vi "PPMS_FreqMeas.vi"(6 "error in (no error)":errorcluster, 7 "Index":i8) -> (0 "error out":errorcluster, 1 "MeasConfig":T1={"Tiempo (sec)"=10.0, "Campo X (T)"=0.025, "Campo Y (T)"=10.0, "Campo Z (T)"=0.025, "Temperatura (K)"=0.025, "Start Frequency (Hz)"=100000.0, "Stop Frequency (Hz)"=1000000.0, "IF Bandwidth"=25.0, "Sweep time(s)"=25.0, "Meas Points"=201, "Power Level (0.0)"=-40.0} {"Campo Z (T)" format="%^.2e"; "Campo Y (T)" format="%^.2e"; "Sweep time(s)" format="%^.2g"; "Temperatura (K)" format="%^.2e"; "Campo X (T)" format="%^.2e"; "Tiempo (sec)" format="%^.2g"; "Start Frequency (Hz)" format="%^.2e"; "IF Bandwidth" format="%^.2e"; "Power Level (0.0)" format="%^.2g"}, 2 "resulting string 1":string="Spectrum from 1.0E+1 Hz to 1.0E+1 Hz, Bandwidth 1.00 Hz, 10 points, Power 10.00 dB", 3 "Cancelled?":bool=TRUE)   [LabVIEW 2017]
doc: "Use this template to create a dialog box. This template polls the state of the buttons on the front panel and does not use events. Use the Dialog Using Events template (not available in Base package) to create a dialog box with event handling."
uses:
  RohdeSchwarz ZNB MeasConfig.ctl
panel:
  in  "Power Level (dB)":dbl=-20.0 format="%.2f"
  in  "Start Frequency (Hz)":dbl=10000000.0 format="%.2p"
  in  "Stop Frequency (Hz)":dbl=10000000000.0 format="%.2p"
  out "MODE":i32(ring) items=["SET&MEAS", "SCAN", "MEASURE ENA3G"]
  in  "IF Bandwidth (Hz)":dbl=50000.0 format="%.2p"
  in  "# Points (2..1601)":u16=5000
  in  "Cancel":bool
  in  "OK":bool
  # "Nov 2020 V1.2  a-sslcdms"
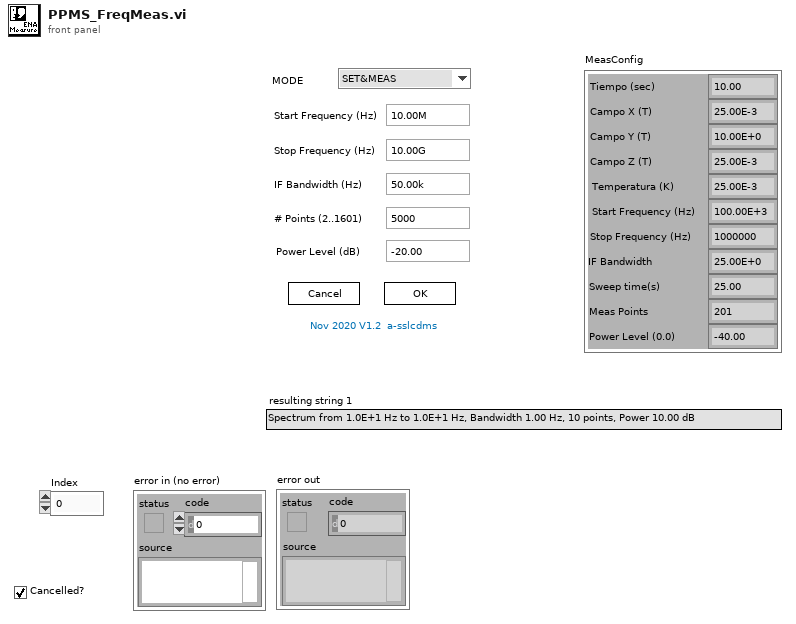
[diagram p1: front panel]
types:
  T1 = typedef "RohdeSchwarz ZNB MeasConfig.ctl" = cluster{"Tiempo (sec)":dbl, "Campo X (T)":dbl, "Campo Y (T)":dbl, "Campo Z (T)":dbl, "Temperatura (K)":dbl, "Start Frequency (Hz)":dbl, "Stop Frequency (Hz)":dbl, "IF Bandwidth":dbl, "Sweep time(s)":dbl, "Meas Points":i32, "Power Level (0.0)":dbl}
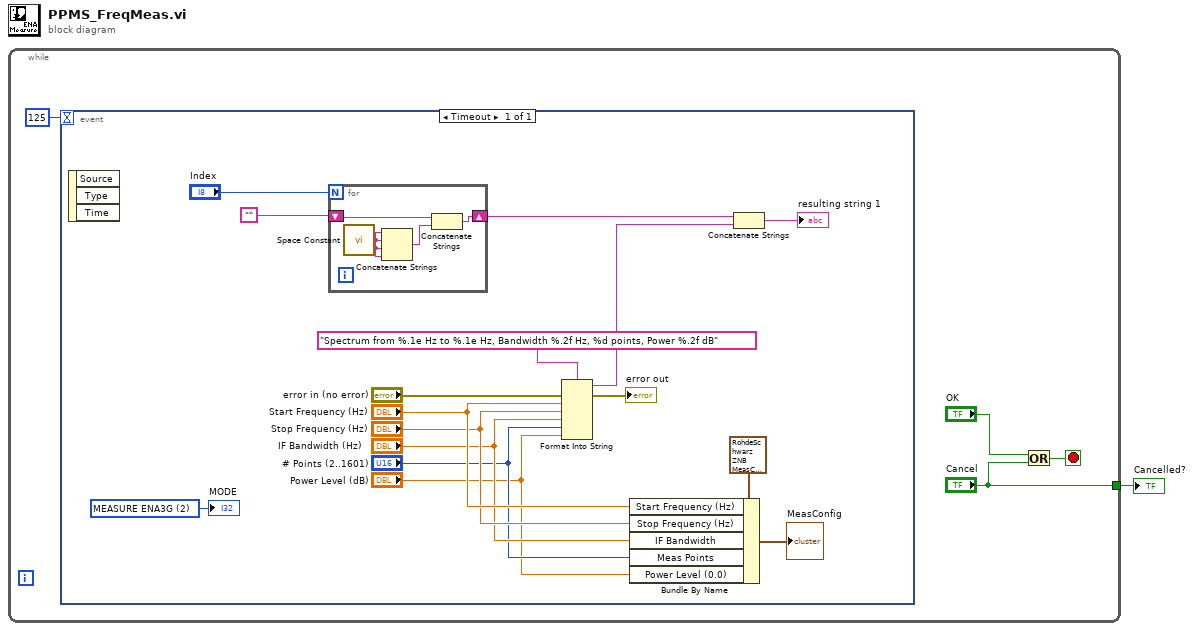
[diagram p0: block diagram]
diagram:
  n1 = while {
    tunnel: ["Cancel"] -> w1
    stop <- w4 stop-if-true
    n2 = event shown="[0] Timeout" {
      selector: _ -> [_]
      dyn-events: _ -> [_]
      timeout: 125 -> [_]
      event Timeout {
        w6 = 2 items=["SET&MEAS", "SCAN", "MEASURE ENA3G"] ("MODE")
        n3 = event-data() -> ()  [unwired: 1 in, 3 out]
        n4 = for {
          N: "Index" -> [_]
          shift-right: [w24] -> w21
          shift-left: "" -> [w23]
          n5 = call <vilib>:"Space Constant.vi"() -> ("String"=w22:string)
          n6 = Concatenate Strings(w22, w22, w22, w22) -> (w25:string)
          n7 = Concatenate Strings(w23, w25) -> (w24:string)
        }
        n8 = Format Into String(format string="Spectrum from %.1e Hz to %.1e Hz, Bandwidth %.2f Hz, %d points, Power %.2f dB", error in="error in (no error)", "Start Frequency (Hz)", "Stop Frequency (Hz)", "IF Bandwidth (Hz)", "# Points (2..1601)", "Power Level (dB)") -> (resulting string=w19:string, error out=→"error out":errorcluster)  [unwired: 1 in]
        n9 = Bundle By Name(cluster=T1 {"Tiempo (sec)"=10.0, "Campo X (T)"=0.025, "Campo Y (T)"=10.0, "Campo Z (T)"=0.025, "Temperatura (K)"=0.025, "Start Frequency (Hz)"=100000.0, "Stop Frequency (Hz)"=1000000.0, "IF Bandwidth"=25.0, "Sweep time(s)"=25.0, "Meas Points"=201, "Power Level (0.0)"=-40.0} ("MeasConfig"), "Start Frequency (Hz)"="Start Frequency (Hz)", "Stop Frequency (Hz)"="Stop Frequency (Hz)", "IF Bandwidth"="IF Bandwidth (Hz)", "Meas Points"="# Points (2..1601)", "Power Level (0.0)"="Power Level (dB)") -> (→"MeasConfig":T1)
        n10 = Concatenate Strings(w21, w19) -> (→"resulting string 1":string)
        "MODE" <- w6
      }
    }
    n11 = Or(x="OK", y="Cancel") -> (x .or. y?=w4:bool)
  }
  "Cancelled?" <- w1
